vi "Open Base System Definition.vi"(8 "error in (no error)":errorcluster) -> (0 "error out":errorcluster, 2 "RAF Custom Device":refnum<k24>, 3 "SystemDefinition":refnum<k24>)   [LabVIEW 2017, in "Switch Scripting System Tests.lvclass"]
uses:
  Switch Scripting System Tests.lvclass
  NationalInstruments.VeriStand.SystemDefinitionAPI
  Scripting/Custom Device/Routing and Faulting Custom Device Settings.ctl
  <userlib>/_OpenG.lib/file/file.llb/Append Path to Root if Relative - Scalar__ogtk.vi
  niveristand-custom-device-testing-tools/VeriStandTestUtilities/VeriStandTestUtilities.lvlib
  Scripting/Switch Scripting.lvlib
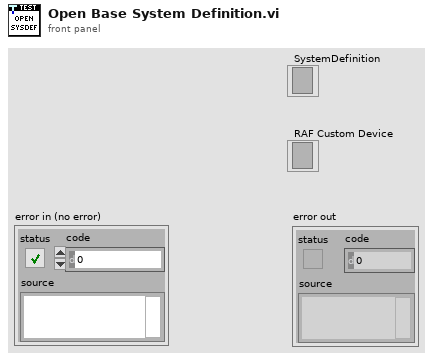
[diagram p1: front panel]
types:
  T1 = typedef "Switch Scripting.lvlib/Routing and Faulting Custom Device Settings.ctl" = cluster{"Name":string}
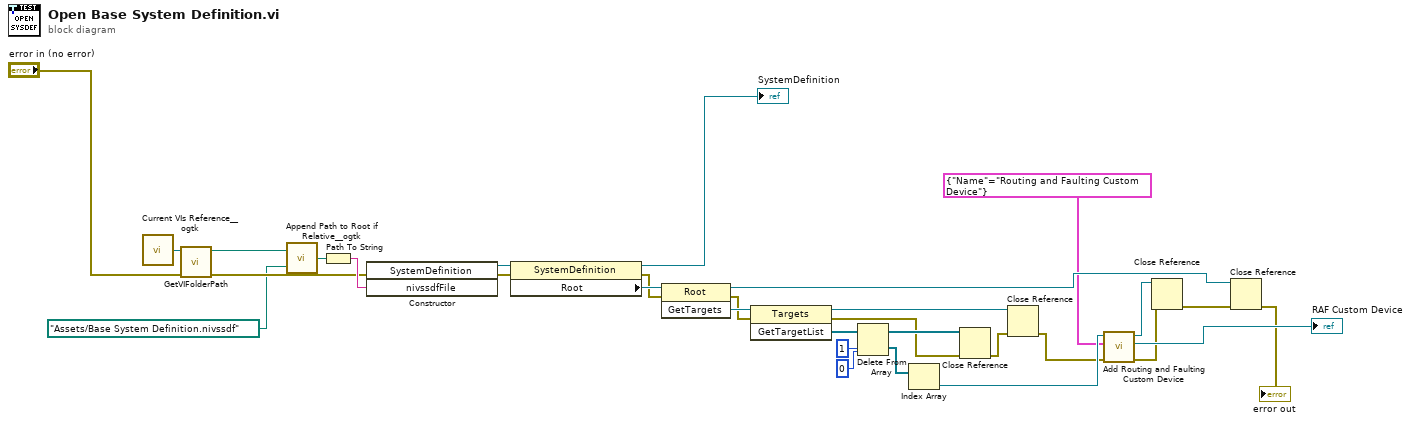
[diagram p0: block diagram]
diagram:
  n1 = call <userlib>:"Current VIs Reference__ogtk.vi"() -> ("Current VI's reference"=w9:refnum<vi>)  [unwired: 5 in]
  n2 = call "GetVIFolderPath.vi"("error in (no error)"="error in (no error)", "VI Reference in"=w9) -> ("error out"=w13:errorcluster, "VI Folder Path out"=w10:path)  [unwired: 8 in]
  n3 = call-poly <userlib>:"Append Path to Root if Relative__ogtk.vi"("Absolute or Relative Path"=path "Assets/Base System Definition.nivssdf", "Root Path"=w10) -> ("Absolute or Appended Path"=w12:path)
  n4 = Path To String(path=w12) -> (string=w15:string)
  n5 = constructor class="SystemDefinition"(error in=w13, "nivssdfFile"=w15) -> (reference out=w16:refnum<k24>, error out=w14:errorcluster)  [unwired: 2 in, 2 out]
  n6 = property class="SystemDefinition"(reference=w16, error in=w14) -> (reference out=→"SystemDefinition":refnum<k24>, error out=w17:errorcluster, "Root"=w18:refnum<k24>)
  n7 = invoke class="Root" method="GetTargets"(reference=w18, error in=w17) -> (reference out=w2:refnum<k24>, error out=w19:errorcluster, "GetTargets"=w20:refnum<k24>)  [unwired: 1 in]
  n8 = invoke class="Targets" method="GetTargetList"(reference=w20, error in=w19) -> (reference out=w27:refnum<k24>, error out=w24:errorcluster, "GetTargetList"=w21:refnum<k24>[])  [unwired: 1 in]
  n9 = Delete From Array(array=w21, length=1, index=0) -> (deleted portion=w28:refnum<k24>[], array with subset deleted=w25:refnum<k24>[])
  n10 = Index Array(array=w28) -> (element=w31:refnum<k24>)  [unwired: 1 in]
  n11 = Close Reference(reference=w25, error in (no error)=w24) -> (error out=w26:errorcluster)
  n12 = Close Reference(reference=w27, error in (no error)=w26) -> (error out=w30:errorcluster)
  n13 = call "Add Routing and Faulting Custom Device.vi"("error in (no error)"=w30, "Settings"=T1 {"Name"="Routing and Faulting Custom Device"}, "Target in"=w31) -> ("error out"=w7:errorcluster, "RAF Custom Device"=→"RAF Custom Device":refnum<k24>, "Target out"=w6:refnum<k24>)  [unwired: 6 in]
  n14 = Close Reference(reference=w6, error in (no error)=w7) -> (error out=w4:errorcluster)
  n15 = Close Reference(reference=w2, error in (no error)=w4) -> (error out=→"error out":errorcluster)
